vi "merFISH_REF_positions_SAVE.vi"(4 "Choice":string, 6 "error in":errorcluster, 9 "REF positions":dbl[][](array[numeric])) -> (0 "error out":errorcluster, 3 "REF positions OUT":dbl[][](array[numeric]))   [LabVIEW 2015]
uses:
  GLOBAL/Global_MAIN.vi
  GLOBAL/Global_ASI_stage.vi
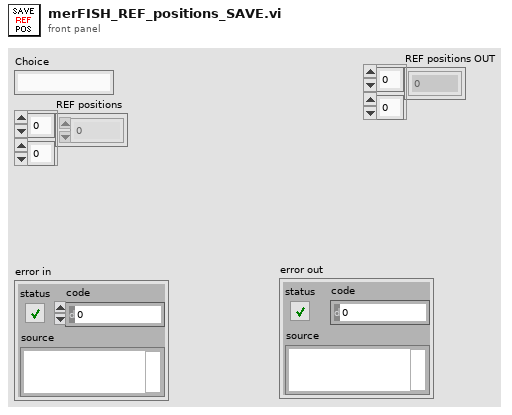
[diagram p1: front panel]
types:
  T1 = enum16{"open", "open or create", "create or replace", "create", "open (read-only)"}
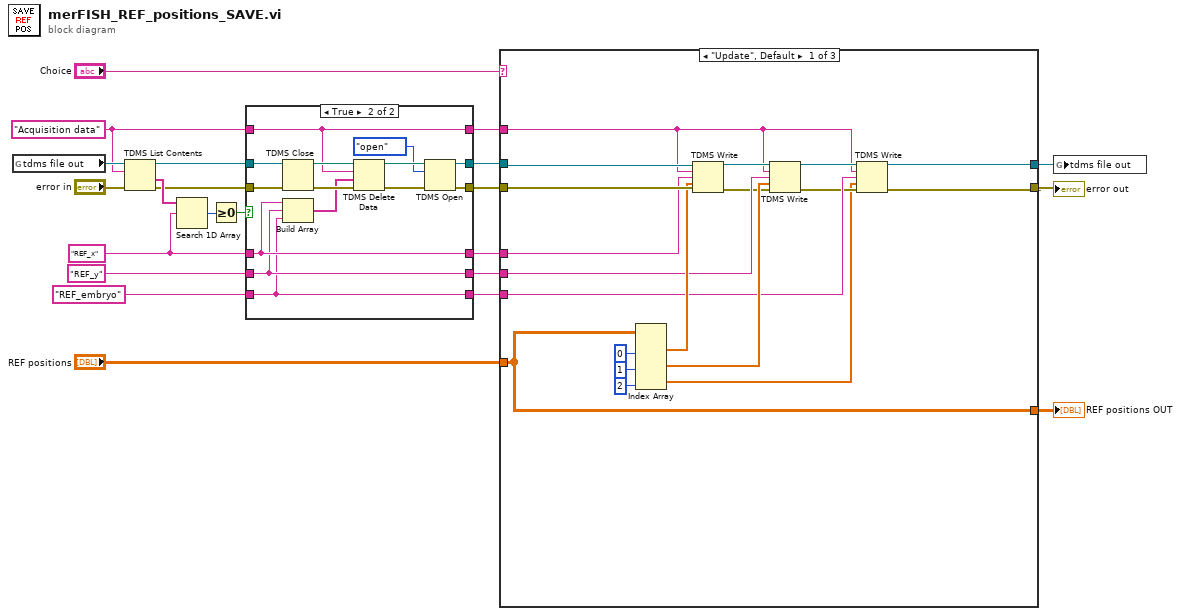
[diagram p0: block diagram]
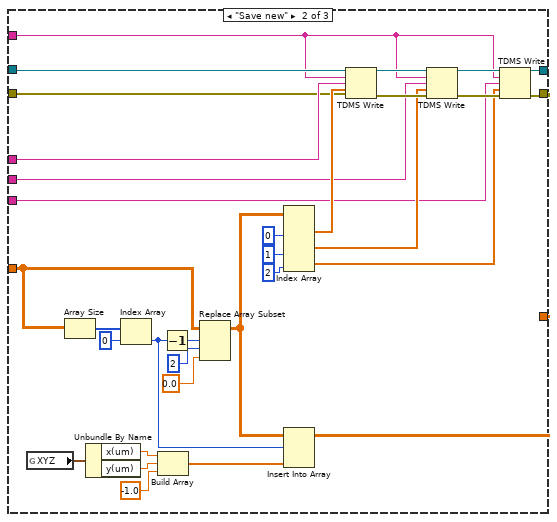
[diagram p3: hidden frame]
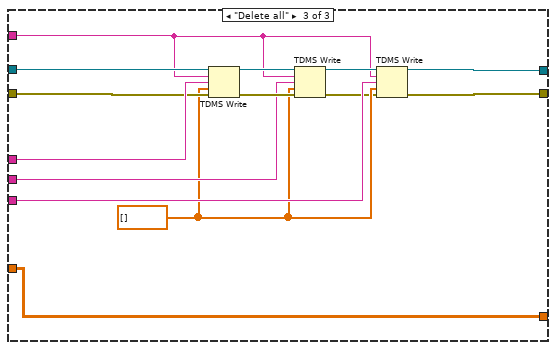
[diagram p4: hidden frame]
diagram:
  w9 = "REF_x"
  w10 = "Acquisition data" ("group name in (Untitled)")
  n1 = global read "Global_MAIN.vi" "tdms file out"() -> (w13:refnum<k34>)
  n2 = TDMS List Contents(4:"error in", 6:w10, 7:w13) -> (0:w8:errorcluster, 1:w14:string[], 3:w11:refnum<k34>)  [unwired: 1 out]
  n3 = Search 1D Array(1D array=w14, element=w9) -> (index of element=w15:i32)  [unwired: 1 in]
  n4 = Greater Or Equal To 0?(x=w15) -> (x >= 0?=w7:bool)
  n5 = case shown="True" w7 {
    tunnel: "REF_y" -> [w25 w31]
    tunnel: [w28 w36] -> w18
    tunnel: [w27 w35] -> w17
    tunnel: w11 -> [w28 w34]
    tunnel: w10 -> [w24 w30]
    tunnel: w9 -> [w26 w32]
    tunnel: w8 -> [w27 w33]
    tunnel: [w26 w32] -> w6
    tunnel: [w25 w31] -> w5
    tunnel: [w24 w30] -> w4
    tunnel: "REF_embryo" -> [w23 w29]
    tunnel: [w23 w29] -> w2
    frame False {
    }
    frame True {
      n6 = TDMS Close(8:w33, 11:w34) -> (0:w41:errorcluster, 3:w42:path)
      n7 = Build Array(w32, w31, w29) -> (w40:string[])
      n8 = TDMS Delete Data(8:w41, 9:w40, 10:w30, 11:w42) -> (0:w38:errorcluster, 3:w39:path)  [unwired: 3 in]
      n9 = TDMS Open(8:w38, 10:T1."open" ("operation (0:open)"), 11:w39) -> (0:w35:errorcluster, 3:w36:refnum<k34>)  [unwired: 4 in]
    }
  }
  n10 = case shown="\"Update\", Default" "Choice" {
    tunnel: [w44 w62 w94] -> w22
    tunnel: "REF positions" -> [w43 w66 w106]
    tunnel: [w43 w63 w106] -> w20
    tunnel: w4 -> [w48 w80 w99]
    tunnel: w6 -> [w59 w92 w107]
    tunnel: [w49 w79 w95] -> w16
    tunnel: w17 -> [w60 w85 w102]
    tunnel: w18 -> [w61 w84 w101]
    tunnel: w5 -> [w54 w89 w103]
    tunnel: w2 -> [w47 w77 w98]
    frame "Update", Default {
      n11 = Index Array(array=w43, index (col) #1=0 ("disabled index (col)"), index (col) #2=1 ("index (col)"), index (col) #3=2 ("index (col)")) -> (element #1=w56:dbl[], element #2=w53:dbl[], element #3=w45:dbl[])  [unwired: 3 in]
      n12 = TDMS Write(0:w61, 5:w48, 7:w59, 9:w56, 11:w60) -> (4:w55:refnum<k34>, 15:w52:errorcluster)  [unwired: 1 in, 2 out]
      n13 = TDMS Write(0:w55, 5:w48, 7:w54, 9:w53, 11:w52) -> (4:w50:refnum<k34>, 15:w46:errorcluster)  [unwired: 1 in, 2 out]
      n14 = TDMS Write(0:w50, 5:w48, 7:w47, 9:w45, 11:w46) -> (4:w49:refnum<k34>, 15:w44:errorcluster)  [unwired: 1 in, 2 out]
    }
    frame "Save new" {
      n15 = global read "Global_ASI_stage.vi" "XYZ"() -> (w71:cluster{"x(um)":dbl, "y(um)":dbl, "z(um)":dbl})
      n16 = Array Size(array=w66) -> (size(s)=w72:i32[])
      n17 = Unbundle By Name(w71) -> ("x(um)"=w70:dbl, "y(um)"=w69:dbl)
      n18 = Index Array(array=w72, index=0) -> (element=w67:i32)
      n19 = Build Array(w70, w69, -1.0 ("element")) -> (w74:dbl[])
      n20 = Decrement(x=w67) -> (x-1=w65:i32)
      n21 = Replace Array Subset(array=w66, new element=0.0 ("new element/subarray"), index (row)=w65, index (col)=2 ("disabled index (col)")) -> (w64:dbl[][])
      n22 = Index Array(array=w64, index (col) #1=0 ("disabled index (col)"), index (col) #2=1 ("index (col)"), index (col) #3=2 ("index (col)")) -> (element #1=w91:dbl[], element #2=w87:dbl[], element #3=w78:dbl[])  [unwired: 3 in]
      n23 = Insert Into Array(array=w64, index (row)=w67, new element=w74) -> (w63:dbl[][])  [unwired: 1 in]
      n24 = TDMS Write(0:w84, 5:w80, 7:w92, 9:w91, 11:w85) -> (4:w86:refnum<k34>, 15:w90:errorcluster)  [unwired: 1 in, 2 out]
      n25 = TDMS Write(0:w86, 5:w80, 7:w89, 9:w87, 11:w90) -> (4:w82:refnum<k34>, 15:w81:errorcluster)  [unwired: 1 in, 2 out]
      n26 = TDMS Write(0:w82, 5:w80, 7:w77, 9:w78, 11:w81) -> (4:w79:refnum<k34>, 15:w62:errorcluster)  [unwired: 1 in, 2 out]
    }
    frame "Delete all" {
      w97 = dbl[] [] ("subarray")
      n27 = TDMS Write(0:w101, 5:w99, 7:w107, 9:w97, 11:w102) -> (4:w105:refnum<k34>, 15:w104:errorcluster)  [unwired: 1 in, 2 out]
      n28 = TDMS Write(0:w105, 5:w99, 7:w103, 9:w97, 11:w104) -> (4:w100:refnum<k34>, 15:w96:errorcluster)  [unwired: 1 in, 2 out]
      n29 = TDMS Write(0:w100, 5:w99, 7:w98, 9:w97, 11:w96) -> (4:w95:refnum<k34>, 15:w94:errorcluster)  [unwired: 1 in, 2 out]
    }
  }
  "error out" <- w22
  "REF positions OUT" <- w20
  n30 = global write "Global_MAIN.vi" "tdms file out"(w16) -> ()
